vi "Parse URL.vi"(8 "error in (no error)":errorcluster, 11 "URL":string) -> (0 "error out":errorcluster, 1 "Path":string, 2 "Port":i32, 3 "Server":string, 5 "Protocol":string)   [LabVIEW 2017, in "Feed.lvclass"]
uses:
  <vilib>/NI_RSS/Feed/Feed.lvclass
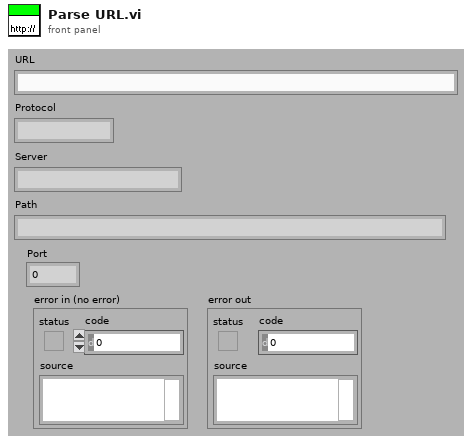
[diagram p1: front panel]
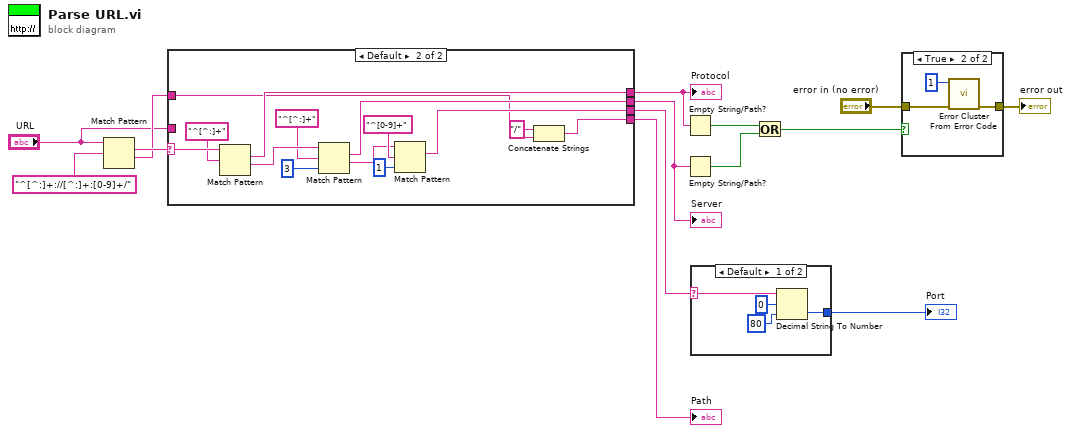
[diagram p0: block diagram]
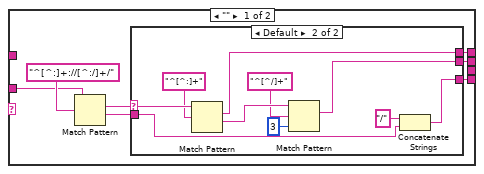
[diagram p2: hidden frame]
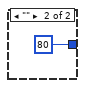
[diagram p5: hidden frame]
diagram:
  n1 = Match Pattern(string="URL", regular expression="^[^:]+://[^:]+:[0-9]+/") -> (match substring=w8:string, after substring=w7:string)  [unwired: 1 in, 2 out]
  n2 = case shown="Default" w8 {
    selector: w8 -> [_ w45]
    tunnel: [w18 w44] -> w2
    tunnel: [w15 w41] -> w3
    tunnel: [_ w40] -> w4
    tunnel: [w16 w37] -> w5
    tunnel: w7 -> [_ w38]
    tunnel: "URL" -> [w20 _]
    frame "" {
      n3 = Match Pattern(string=w20, regular expression="^[^:]+://[^:/]+/") -> (match substring=w19:string, after substring=w17:string)  [unwired: 1 in, 2 out]
      n4 = case shown="Default" w19 {
        selector: w19 -> [_ w31]
        tunnel: [_ w30] -> w18
        tunnel: w17 -> [_ w23]
        tunnel: [_ w24] -> w16
        tunnel: [_ w22] -> w15
        frame "" {
        }
        frame Default {
          n5 = Match Pattern(string=w31, regular expression="^[^:]+") -> (match substring=w30:string, after substring=w29:string)  [unwired: 1 in, 2 out]
          n6 = Match Pattern(string=w29, regular expression="^[^/]+", offset (0)=3) -> (match substring=w22:string)  [unwired: 3 out]
          n7 = Concatenate Strings("/" ("string"), w23) -> (w24:string)
        }
      }
    }
    frame Default {
      n8 = Match Pattern(string=w45, regular expression="^[^:]+") -> (match substring=w44:string, after substring=w43:string)  [unwired: 1 in, 2 out]
      n9 = Match Pattern(string=w43, regular expression="^[^:]+", offset (0)=3) -> (match substring=w41:string, after substring=w33:string)  [unwired: 2 out]
      n10 = Match Pattern(string=w33, regular expression="^[0-9]+", offset (0)=1) -> (match substring=w40:string)  [unwired: 3 out]
      n11 = Concatenate Strings("/" ("string"), w38) -> (w37:string)
    }
  }
  "Protocol" <- w2
  "Server" <- w3
  "Path" <- w5
  n12 = Empty String/Path?(string/path=w2) -> (empty?=w13:bool)
  n13 = Empty String/Path?(string/path=w3) -> (empty?=w12:bool)
  n14 = case shown="Default" w4 {
    selector: w4 -> [w47 _]
    tunnel: [w49 80 ("offset past number")] -> w14
    frame Default {
      n15 = Decimal String To Number(string=w47, offset=0, default (0L)=80 ("default (0 I32)")) -> (number=w49:i32)  [unwired: 1 out]
    }
    frame "" {
    }
  }
  "Port" <- w14
  n16 = Or(x=w13, y=w12) -> (x .or. y?=w11:bool)
  n17 = case shown="True" w11 {
    tunnel: "error in (no error)" -> [w51 w53]
    tunnel: [w51 w52] -> w10
    frame False {
    }
    frame True {
      n18 = call <vilib>:"Error Cluster From Error Code.vi"("error in (no error)"=w53, "error code (0)"=1) -> ("error out"=w52:errorcluster)  [unwired: 1 in, 6 out]
    }
  }
  "error out" <- w10
